vi "Make_Saw_Direct.vi"(1 "N_steps_1":i32 min=0 step=1) -> (0 "SawDirectWaveform":dbl[](array[numeric]))   [LabVIEW 2019]
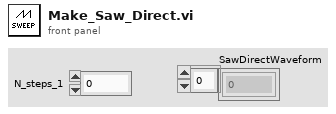
[diagram p1: front panel]
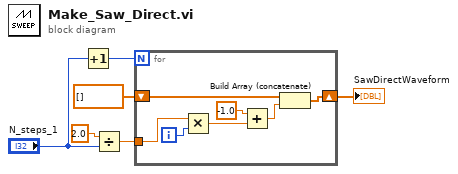
[diagram p0: block diagram]
diagram:
  n1 = Increment(x="N_steps_1") -> (x+1=w3:i32)
  n2 = Divide(x=2.0, y="N_steps_1") -> (x/y=w5:dbl)
  n3 = for {
    N: w3 -> [_]
    tunnel: w5 -> [w11]
    shift-right: [w8] -> w1
    shift-left: dbl[] [] -> [w9]
    i -> [w12]
    n4 = Multiply(x=w11, y=w12) -> (x*y=w10:dbl)
    n5 = Add(x=-1.0, y=w10) -> (x+y=w7:dbl)
    n6 = Build Array (concatenate)(w9, w7) -> (w8:dbl[])
  }
  "SawDirectWaveform" <- w1
